vi "Brain.vi"() -> ()   [LabVIEW 2017]
uses:
  <vilib>/OPCUA/controls/NodeId.ctl
  <vilib>/OPCUA/controls/Write Status.ctl
  <vilib>/Utility/file.llb/Read Delimited Spreadsheet (string).vi
  <vilib>/Utility/file.llb/Write Delimited Spreadsheet (string).vi
  <vilib>/OPCUA/client/Multiple Write Double Array.vi
  <vilib>/Utility/file.llb/Write Delimited Spreadsheet (DBL).vi
  <resource>/objmgr/ni.dex.rc
  <vilib>/OPCUA/NI OPC UA Client.lvlib
panel:
  in  "VFD Stop":bool
  in  "Shutdown":bool
  out "Remote VI Error Messages":string
  in  "Node Status":u16
  in  "Time Stamp":timestamp
  out "Error Out":errorcluster
  in  "Stop DAQ":bool
  out "DAQ?":bool
  out "Available Elements for Reading":i32
  out "Number of Disconnections":u32
  out "System Loop Time (ms)":u32
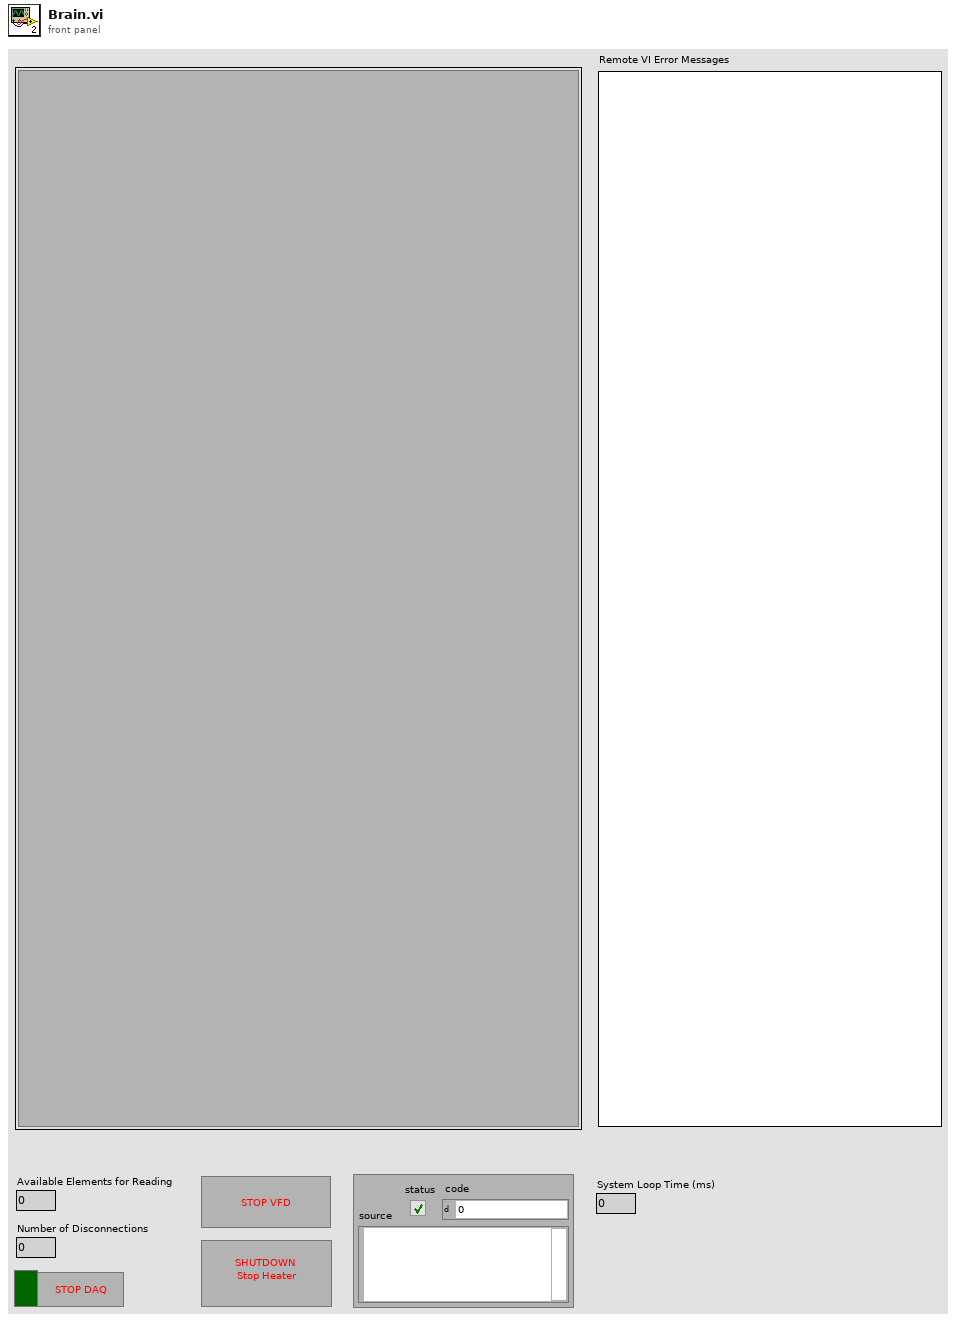
[diagram p1: front panel]
types:
  T1 = typedef "OPC UA Client Refnum.ctl" = refnum<k21>
  T2 = typedef "NodeId.ctl" = string
  T3 = typedef "Write Status.ctl" = u32
  T4 = cluster{"node ID":T2, "value":dbl[], "timestamp (current time)":timestamp, "node status":T3}
  T5 = cluster{"node ID":T2, "value":dbl[], "timestamp (current time)":timestamp, "node status":T3}[]
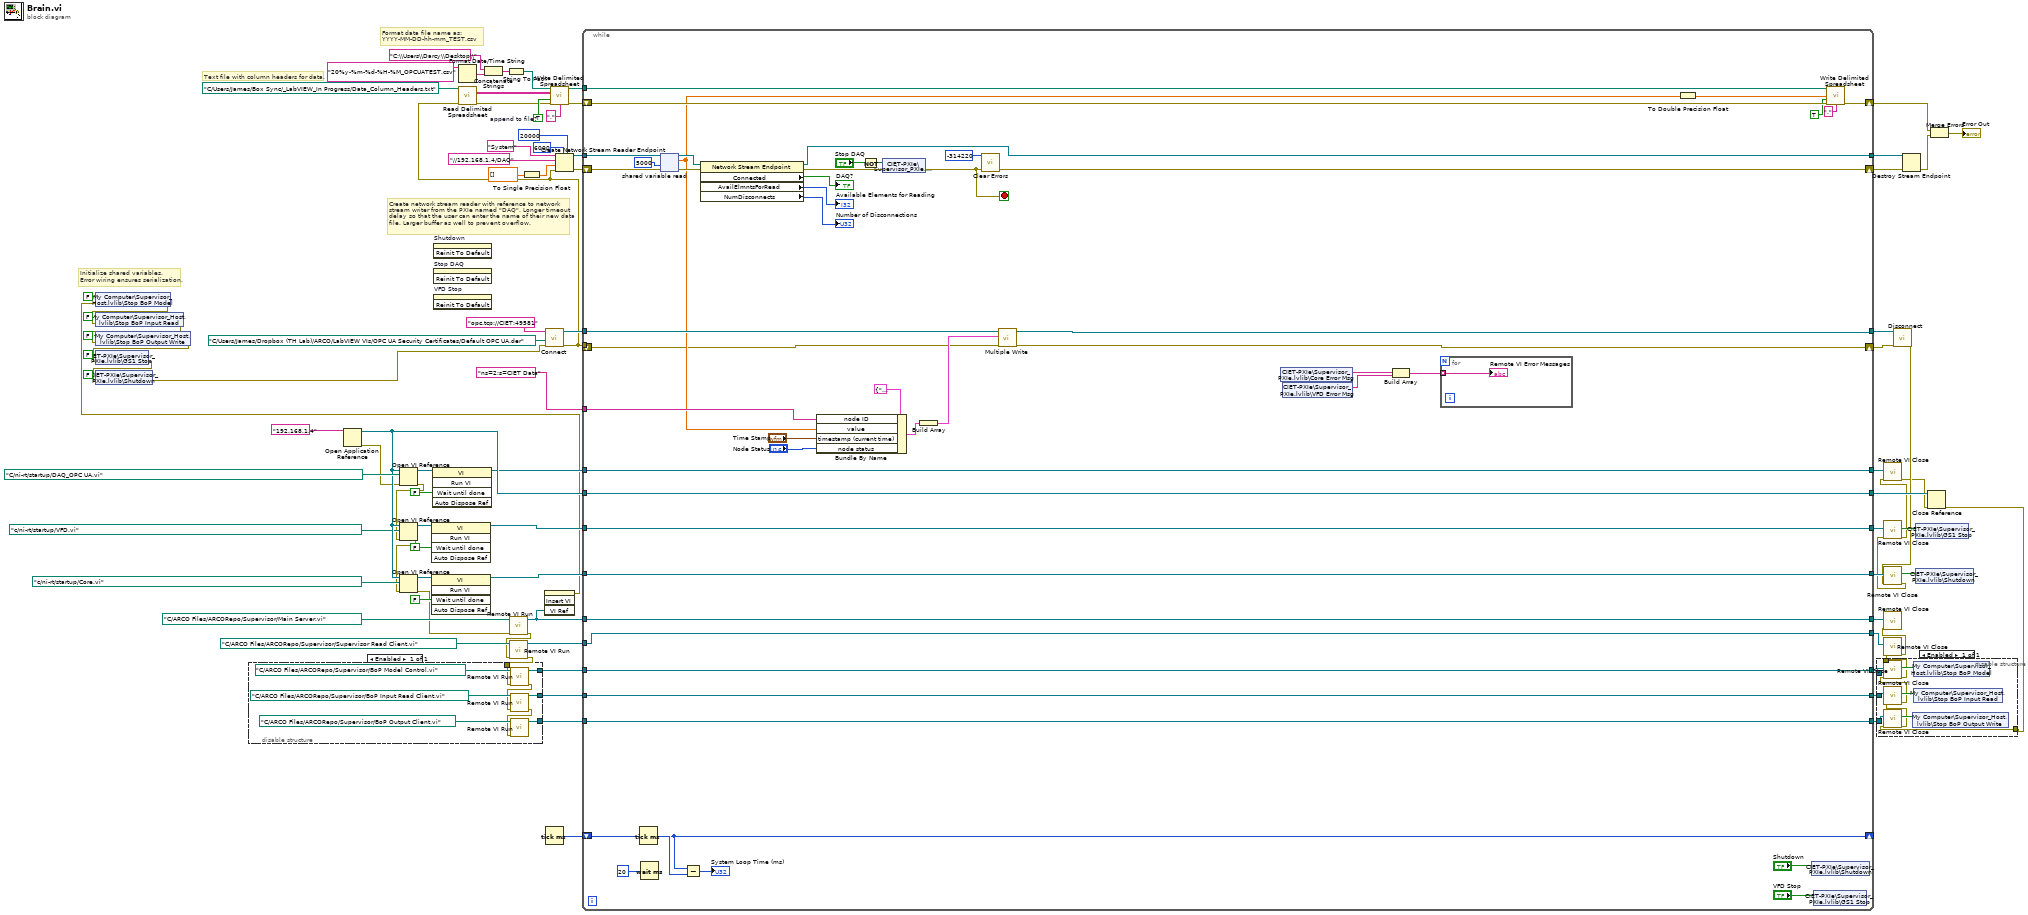
[diagram p0: block diagram]
diagram:
  w76 = TRUE  # append to file?
  # "Initialize shared variables.\nError wiring ensures serialization."
  # "Format data file name as:\nYYYY-MM-DD-hh-mm_TEST.csv"
  # "Create network stream reader with reference to network\nstream writer from the PXIe named \"DAQ\". Longer timeout\ndelay so that the user can enter the name of their new data\nfile. Larger buffer as well to prevent overflow."
  # "Text file with column headers for data."
  n1 = Open Application Reference(11:"192.168.1.4" ("machine name (\"\":  open local reference)")) -> (0:w14:errorcluster, 3:w49:refnum<vi>)  [unwired: 3 in]
  n2 = Open VI Reference(application reference (local)=w49, vi path=path "C:/ni-rt/startup/DAQ_OPC UA.vi", error in (no error)=w14) -> (vi reference=w46:refnum<vi>, error out=w13:errorcluster)  [unwired: 3 in]
  n3 = Open VI Reference(application reference (local)=w49, vi path=path "c:/ni-rt/startup/VFD.vi", error in (no error)=w13) -> (vi reference=w44:refnum<vi>, error out=w12:errorcluster)  [unwired: 3 in]
  n4 = Open VI Reference(application reference (local)=w49, vi path=path "c:/ni-rt/startup/Core.vi", error in (no error)=w12) -> (vi reference=w42:refnum<vi>, error out=w11:errorcluster)  [unwired: 3 in]
  n5 = invoke class="VI" method="Run VI"(reference=w44, "Wait until done"=FALSE ("Wait Until Done")) -> (reference out=w43:refnum<vi>)  [unwired: 3 in, 4 out]
  n6 = invoke class="VI" method="Run VI"(reference=w42, "Wait until done"=FALSE ("Wait Until Done")) -> (reference out=w41:refnum<vi>)  [unwired: 3 in, 4 out]
  n7 = invoke class="VI" method="Run VI"(reference=w46, "Wait until done"=FALSE ("Wait Until Done")) -> (reference out=w45:refnum<vi>)  [unwired: 3 in, 4 out]
  n8 = invoke on="Shutdown" class="Bool (strict)" method="Reinit To Default"() -> ()  [unwired: 3 in, 3 out]
  n9 = invoke on="Stop DAQ" class="Bool (strict)" method="Reinit To Default"() -> ()  [unwired: 3 in, 3 out]
  n10 = invoke on="VFD Stop" class="Bool (strict)" method="Reinit To Default"() -> ()  [unwired: 3 in, 3 out]
  n11 = Format Date/Time String(time format string (%c)="20%y-%m-%d-%H-%M_OPCUATEST.csv") -> (date/time string=w66:string)  [unwired: 2 in]
  n12 = Concatenate Strings("C:\\Users\\Darcy\\Desktop\\" ("string"), w66) -> (w68:string)
  n13 = String To Path(string=w68) -> (path=w65:path)
  n14 = call "Remote VI Run.vi"("error in (no error)"=w11, "VI Path"=path "C:/ARCO Files/ARCORepo/Supervisor/Main Server.vi" ("vi path")) -> ("error out"=w9:errorcluster, "VI Reference"=w51:refnum<vi>)  [unwired: 8 in]
  n15 = call "Remote VI Run.vi"("error in (no error)"=w9, "VI Path"=path "C:/ARCO Files/ARCORepo/Supervisor/Supervisor Read Client.vi" ("vi path")) -> ("error out"=w10:errorcluster, "VI Reference"=w34:refnum<vi>)  [unwired: 8 in]
  n16 = disable-structure shown="Enabled" {
    disable-tunnel: [w95] -> w32
    disable-tunnel: [w94] -> w30
    disable-tunnel: [w93] -> w28
    disable-tunnel: w10 -> [w92]
    frame Enabled {
      n17 = call "Remote VI Run.vi"("error in (no error)"=w92, "VI Path"=path "C:/ARCO Files/ARCORepo/Supervisor/BoP Model Control.vi" ("vi path")) -> ("error out"=w91:errorcluster, "VI Reference"=w95:refnum<vi>)  [unwired: 8 in]
      n18 = call "Remote VI Run.vi"("error in (no error)"=w91, "VI Path"=path "C:/ARCO Files/ARCORepo/Supervisor/BoP Input Read Client.vi" ("vi path")) -> ("error out"=w90:errorcluster, "VI Reference"=w94:refnum<vi>)  [unwired: 8 in]
      n19 = call "Remote VI Run.vi"("error in (no error)"=w90, "VI Path"=path "C:/ARCO Files/ARCORepo/Supervisor/BoP Output Client.vi" ("vi path")) -> ("VI Reference"=w93:refnum<vi>)  [unwired: 8 in, 1 out]
    }
  }
  n20 = To Single Precision Float(number=dbl[] []) -> (single precision float=w87:sgl[])
  n21 = invoke on="Sub Panel" class="SubPnl" method="Insert VI"("VI Ref"=w51) -> (error out=w1:errorcluster)  [unwired: 3 in, 3 out]
  n22 = shared-variable "My Computer\\Supervisor_Host.lvlib\\Stop BoP Model"(FALSE ("Stop BoP Model"), error in=w1) -> (error out=w25:errorcluster)
  n23 = shared-variable "My Computer\\Supervisor_Host.lvlib\\Stop BoP Input Read"(FALSE ("Stop BoP Input Read"), error in=w25) -> (error out=w24:errorcluster)
  n24 = shared-variable "My Computer\\Supervisor_Host.lvlib\\Stop BoP Output Write"(FALSE ("Stop BoP Output Write"), error in=w24) -> (error out=w23:errorcluster)
  n25 = shared-variable "CIET-PXIe\\Supervisor_PXIe.lvlib\\GS1 Stop"(FALSE ("GS1 Stop"), error in=w23) -> (error out=w22:errorcluster)
  n26 = shared-variable "CIET-PXIe\\Supervisor_PXIe.lvlib\\Shutdown"(FALSE ("Shutdown"), error in=w22) -> (error out=w21:errorcluster)
  n27 = call <vilib>:"Connect.vi"("error in (no error)"=w21, "client certificate file"=path "C:/Users/James/Dropbox (TH Lab)/ARCO/LabVIEW VIs/OPC UA Security Certificates/Default OPC UA.der", "server endpoint URL"="opc.tcp://CIET:49581") -> ("error out"=w15:errorcluster, "OPC UA client refnum out"=w61:T1)  [unwired: 6 in, 1 out]
  n28 = call-poly <vilib>:"Read Delimited Spreadsheet.vi"("file path (dialog if empty)"=path "C:/Users/James/Box Sync/_LabVIEW_In Progress/Data_Column_Headers.txt", "error in (no error)"=w15) -> ("all rows"=w79:string[][], "error out"=w74:errorcluster)  [unwired: 8 in, 4 out]
  n29 = Tick Count (ms)() -> (millisecond timer value=w64:u32)
  n30 = call-poly <vilib>:"Write Delimited Spreadsheet.vi"("file path (dialog if empty)"=w65, "2D data"=w79, "append to file? (new file:F)"=w76, "error in (no error)"=w74, "delimiter (\\t)"=",") -> ("new file path (Not A Path if cancelled)"=w75:path, "error out"=w73:errorcluster)  [unwired: 9 in]
  n31 = Create Network Stream Reader Endpoint(5:20000 ("timeout in ms (-1)"), 7:6000 ("reader buffer size"), 8:w15, 9:w87, 10:"//192.168.1.4/DAQ" ("writer url"), 11:"System" ("reader name")) -> (0:w84:errorcluster, 3:w83:refnum<k21>)  [unwired: 1 in]
  n32 = while {
    shift-right: [w137] -> w82
    shift-left: w84 -> [w145]
    tunnel: w83 -> [w146]
    tunnel: [w136] -> w81
    tunnel: w75 -> [w132]
    shift-right: [w130] -> w72
    shift-left: w73 -> [w131]
    shift-right: [w125] -> _
    shift-left: w64 -> [w126]
    tunnel: w61 -> [w120]
    tunnel: w15 -> [_]
    tunnel: "ns=2;s=CIET Data" -> [w119]
    tunnel: [w102] -> w59
    tunnel: w45 -> [w118]
    tunnel: [w118] -> w56
    tunnel: w49 -> [w117]
    tunnel: [w117] -> w55
    tunnel: w43 -> [w116]
    tunnel: [w116] -> w54
    tunnel: w41 -> [w115]
    tunnel: [w115] -> w53
    tunnel: w51 -> [w114]
    tunnel: [w114] -> w52
    tunnel: w34 -> [w106]
    tunnel: [w106] -> w33
    tunnel: w32 -> [w105]
    tunnel: [w105] -> w31
    tunnel: w30 -> [w104]
    tunnel: [w104] -> w29
    tunnel: w28 -> [w103]
    tunnel: [w103] -> w27
    shift-right: [w99] -> w58
    shift-left: _ -> [w100]
    stop <- w135 stop-if-true
    n33 = Tick Count (ms)() -> (millisecond timer value=w125:u32)
    n34 = Wait (ms)(milliseconds to wait=u32 20) -> ()  [unwired: 1 out]
    n35 = shared-variable-read(w146, w145, 5000 ("timeout ms (-1)")) -> (w142:refnum<k21>, w140:errorcluster, w101:sgl[])  [unwired: 1 out]
    n36 = Subtract(x=w125, y=w126) -> (x-y=→"System Loop Time (ms)":u32)
    n37 = property class="Network Stream Endpoint"(reference=w142, error in=w140) -> (reference out=w136:refnum<k21>, error out=w141:errorcluster, "Connected"=→"DAQ?":bool, "AvailElmntsForRead"=→"Available Elements for Reading":i32, "NumDisconnects"=→"Number of Disconnections":u32)
    n38 = Bundle By Name(cluster=T4 {"node ID"="", "value"=[], "timestamp (current time)"=timestamp(0 s since 1904-01-01), "node status"=0} ("request"), "node ID"=w119, "value"=w101, "timestamp (current time)"="Time Stamp", "node status"="Node Status") -> (w122:T4)
    n39 = Not(x="Stop DAQ") -> (.not. x?=w144:bool)
    n40 = shared-variable "CIET-PXIe\\Supervisor_PXIe.lvlib\\DAQ?"(w144, error in=w141) -> (error out=w135:errorcluster)
    n41 = Build Array(w122) -> (w121:T5)
    n42 = call <vilib>:"Clear Errors.vi"("error in (no error)"=w135, "specific error code to clear (0: all)"=-314220) -> ("error out"=w137:errorcluster)  [unwired: 4 in, 1 out]
    n43 = call-poly <vilib>:"Multiple Write.vi"("error in (no error)"=w100, "requests"=w121, "OPC UA client refnum in"=w120) -> ("error out"=w99:errorcluster, "OPC UA client refnum out"=w102:T1)  [unwired: 5 in, 2 out]
    n44 = shared-variable "CIET-PXIe\\Supervisor_PXIe.lvlib\\Core Error Msg"() -> (w113:string)  [unwired: 1 in, 1 out]
    n45 = shared-variable "CIET-PXIe\\Supervisor_PXIe.lvlib\\VFD Error Msg"() -> (w112:string)  [unwired: 1 in, 1 out]
    n46 = Build Array(w113, w112) -> (w111:string[])
    n47 = for {
      tunnel: w111 -> [w149] mode=indexing
      "Remote VI Error Messages" <- w149
    }
    n48 = To Double Precision Float(number=w101) -> (double precision float=w127:dbl[])
    n49 = shared-variable "CIET-PXIe\\Supervisor_PXIe.lvlib\\Shutdown"("Shutdown") -> ()  [unwired: 1 in, 1 out]
    n50 = shared-variable "CIET-PXIe\\Supervisor_PXIe.lvlib\\GS1 Stop"("VFD Stop") -> ()  [unwired: 1 in, 1 out]
    n51 = call-poly <vilib>:"Write Delimited Spreadsheet.vi"("file path (dialog if empty)"=w132, "1D data"=w127, "append to file? (new file:F)"=TRUE, "error in (no error)"=w131, "delimiter (\\t)"="," ("delimiter (\\t)")) -> ("error out"=w130:errorcluster)  [unwired: 9 in, 1 out]
  }
  n52 = call <vilib>:"Disconnect.vi"("error in (no error)"=w58, "OPC UA client refnum in"=w59) -> ("error out"=w8:errorcluster)  [unwired: 9 in]
  n53 = call "Remote VI Close.vi"("error in (no error)"=w8, "reference"=w53) -> ("error out"=w7:errorcluster, "SubVI Stop"=w37:bool)  [unwired: 8 in]
  n54 = call "Remote VI Close.vi"("error in (no error)"=w7, "reference"=w54) -> ("error out"=w6:errorcluster, "SubVI Stop"=w26:bool)  [unwired: 8 in]
  n55 = call "Remote VI Close.vi"("error in (no error)"=w6, "reference"=w56) -> ("error out"=w5:errorcluster)  [unwired: 8 in, 1 out]
  n56 = Destroy Stream Endpoint(8:w82, 11:w81) -> (0:w71:errorcluster)
  n57 = shared-variable "CIET-PXIe\\Supervisor_PXIe.lvlib\\GS1 Stop"(w26) -> ()  [unwired: 1 in, 1 out]
  n58 = shared-variable "CIET-PXIe\\Supervisor_PXIe.lvlib\\Shutdown"(w37) -> ()  [unwired: 1 in, 1 out]
  n59 = Close Reference(reference=w55, error in (no error)=w5) -> (error out=w4:errorcluster)
  n60 = disable-structure shown="Enabled" {
    disable-tunnel: w31 -> [w159]
    disable-tunnel: w29 -> [w158]
    disable-tunnel: w27 -> [w157]
    disable-tunnel: w4 -> [w153]
    disable-tunnel: [w150] -> w3
    frame Enabled {
      n61 = call "Remote VI Close.vi"("error in (no error)"=w153, "reference"=w157) -> ("error out"=w152:errorcluster, "SubVI Stop"=w156:bool)  [unwired: 8 in]
      n62 = call "Remote VI Close.vi"("error in (no error)"=w152, "reference"=w158) -> ("error out"=w151:errorcluster, "SubVI Stop"=w154:bool)  [unwired: 8 in]
      n63 = call "Remote VI Close.vi"("error in (no error)"=w151, "reference"=w159) -> ("error out"=w150:errorcluster, "SubVI Stop"=w155:bool)  [unwired: 8 in]
      n64 = shared-variable "My Computer\\Supervisor_Host.lvlib\\Stop BoP Output Write"(w156) -> ()  [unwired: 1 in, 1 out]
      n65 = shared-variable "My Computer\\Supervisor_Host.lvlib\\Stop BoP Model"(w155) -> ()  [unwired: 1 in, 1 out]
      n66 = shared-variable "My Computer\\Supervisor_Host.lvlib\\Stop BoP Input Read"(w154) -> ()  [unwired: 1 in, 1 out]
    }
  }
  n67 = call "Remote VI Close.vi"("error in (no error)"=w3, "reference"=w33) -> ("error out"=w2:errorcluster)  [unwired: 8 in, 1 out]
  n68 = call "Remote VI Close.vi"("error in (no error)"=w2, "reference"=w52) -> ()  [unwired: 8 in, 2 out]
  n69 = Merge Errors(w72, w71) -> (→"Error Out":errorcluster)
